vi "Receive Interface Status.vi"(8 "error in (no error)":errorcluster, 11 "Stream in":refnum<class "Stream.lvclass">) -> (0 "error out":errorcluster, 3 "Stream out":refnum<class "Stream.lvclass">)   [LabVIEW 2018, in "Stream.lvclass"]
uses:
  Stream.lvclass
  Interface/Interface.lvclass
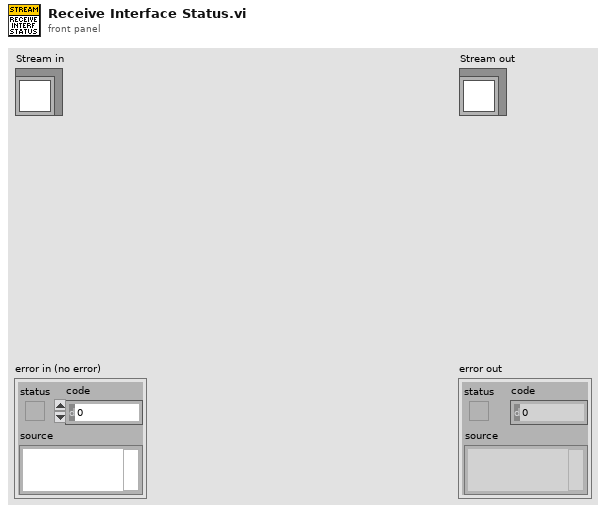
[diagram p1: front panel]
types:
  T1 = cluster{"Current Temperature":i16, "Temperatue Status":string}
  T2 = cluster{"Initialization":bool, "Serial Number":u16}
  T3 = cluster{"Exposure Time":sgl, "Pre-amp gain":u8, "Readout Rate":u8, "EM Mode":u8, "EM Gain":u16, "Binning":u16, "Initial Line":u16, "Initial Cloumn":u16, "Final Line":u16, "Final Column":u16, "Kinetic Series Length":u32, "Shutter Mode":u8, "Cooler ON/OFF":u16, "Temperature":i8, "Image Name":string, "Image Path":string, "#Images":u32, "Trigger":u16}
  T4 = cluster{"CUBE_EXPOSURE_TIME":sgl, "CUBES_DONE":u16, "LAST_IMAGE_NAME":string, "DISK_SPACE":u16, "FRAMES_DONE":u16, "CCD_STATUS":string, "CURRENT_TEMPERATURE":i16, "TEMPERATURE_STATUS":string, "FRAME_EXPOSURE_TIME":u16, "CCD_ON_OFF":bool, "SERIAL_NUMBER":u16, "ACQUIRING":bool}
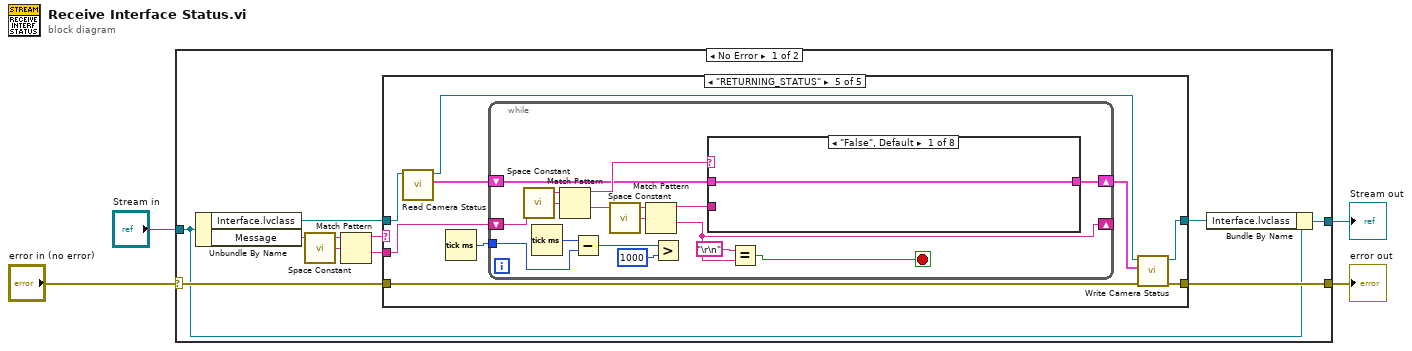
[diagram p0: block diagram]
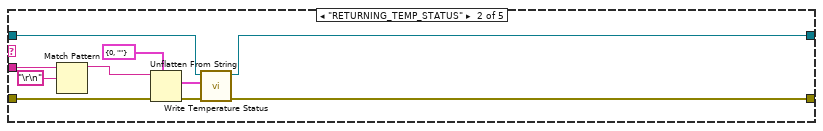
[diagram p3: hidden frame]
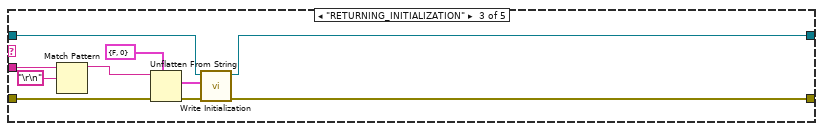
[diagram p4: hidden frame]
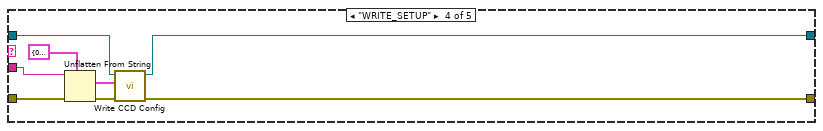
[diagram p5: hidden frame]
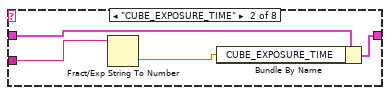
[diagram p6: hidden frame]
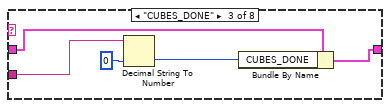
[diagram p7: hidden frame]
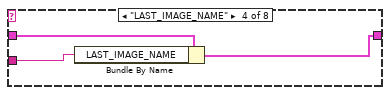
[diagram p8: hidden frame]
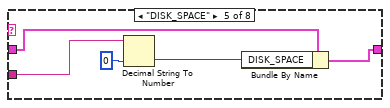
[diagram p9: hidden frame]
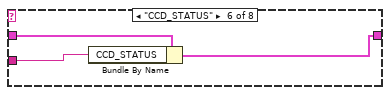
[diagram p10: hidden frame]
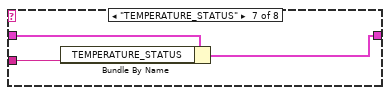
[diagram p11: hidden frame]
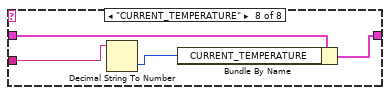
[diagram p12: hidden frame]
diagram:
  n1 = case shown="No Error" "error in (no error)" {
    selector: "error in (no error)" -> [w8 w98]
    tunnel: [w9 w98] -> w3
    tunnel: [w6 w97] -> w1
    tunnel: "Stream in" -> [w7 w97]
    frame No Error {
      n2 = Unbundle By Name(w7) -> ("Interface.lvclass"=w11:refnum<class "Interface.lvclass">, "Message"=w10:string)
      n3 = call <vilib>:"Space Constant.vi"() -> ("String"=w14:string)
      n4 = Match Pattern(string=w10, regular expression=w14) -> (before substring=w5:string, after substring=w13:string)  [unwired: 1 in, 2 out]
      n5 = case shown="\"RETURNING_STATUS\"" w5 {
        tunnel: w13 -> [_ w19 w28 w39 w45]
        tunnel: [w16 w26 w33 w41 w49] -> w12
        tunnel: w11 -> [w16 w25 w34 w40 w52]
        tunnel: [w15 w21 w32 w42 w48] -> w9
        tunnel: w8 -> [w15 w20 w31 w43 w47]
        frame "False", Default {
        }
        frame "RETURNING_TEMP_STATUS" {
          n6 = Match Pattern(string=w19, regular expression="\r\n") -> (before substring=w17:string)  [unwired: 1 in, 3 out]
          n7 = Unflatten From String(type=T1 {"Current Temperature"=0, "Temperatue Status"=""} ("Temperature Status"), binary string=w17, error in (no error)=w20) -> (value=w23:T1, error out=w24:errorcluster)  [unwired: 2 in, 1 out]
          n8 = call "Write Temperature Status.vi"("error in (no error)"=w24, "Temperature Status"=w23, "Interface in"=w25) -> ("error out"=w21:errorcluster, "Interface out"=w26:refnum<class "Interface.lvclass">)  [unwired: 7 in]
        }
        frame "RETURNING_INITIALIZATION" {
          n9 = Match Pattern(string=w28, regular expression="\r\n") -> (before substring=w27:string)  [unwired: 1 in, 3 out]
          n10 = Unflatten From String(type=T2 {"Initialization"=FALSE, "Serial Number"=0} ("Initialization"), binary string=w27, error in (no error)=w31) -> (value=w30:T2, error out=w36:errorcluster)  [unwired: 2 in, 1 out]
          n11 = call "Write Initialization.vi"("error in (no error)"=w36, "Initialization"=w30, "Interface in"=w34) -> ("error out"=w32:errorcluster, "Interface out"=w33:refnum<class "Interface.lvclass">)  [unwired: 7 in]
        }
        frame "WRITE_SETUP" {
          n12 = Unflatten From String(type=T3 {"Exposure Time"=0.0, "Pre-amp gain"=0, "Readout Rate"=0, "EM Mode"=0, "EM Gain"=0, "Binning"=0, "Initial Line"=0, "Initial Cloumn"=0, "Final Line"=0, "Final Column"=0, "Kinetic Series Length"=0, "Shutter Mode"=0, "Cooler ON/OFF"=0, "Temperature"=0, "Image Name"="", "Image Path"="", "#Images"=0, "Trigger"=0} ("CCD Config"), binary string=w39, error in (no error)=w43) -> (value=w38:T3, error out=w44:errorcluster)  [unwired: 2 in, 1 out]
          n13 = call "Write CCD Config.vi"("error in (no error)"=w44, "CCD Config"=w38, "Interface in"=w40) -> ("error out"=w42:errorcluster, "Interface out"=w41:refnum<class "Interface.lvclass">)  [unwired: 7 in]
        }
        frame "RETURNING_STATUS" {
          n14 = call "Read Camera Status.vi"("Interface in"=w52) -> ("Camera Status"=w50:T4, "Interface out"=w51:refnum<class "Interface.lvclass">)  [unwired: 8 in, 1 out]
          n15 = Tick Count (ms)() -> (millisecond timer value=w46:u32)
          n16 = while {
            shift-right: [w65] -> w53
            shift-left: w50 -> [w64]
            shift-right: [w60] -> _
            shift-left: w45 -> [w67]
            tunnel: w46 -> [w57]
            stop <- w54 stop-if-true
            n17 = call <vilib>:"Space Constant.vi"() -> ("String"=w68:string)
            n18 = Tick Count (ms)() -> (millisecond timer value=w58:u32)
            n19 = Match Pattern(string=w67, regular expression=w68) -> (before substring=w66:string, after substring=w62:string)  [unwired: 1 in, 2 out]
            n20 = Subtract(x=w58, y=w57) -> (x-y=w56:u32)
            n21 = call <vilib>:"Space Constant.vi"() -> ("String"=w63:string)
            n22 = Match Pattern(string=w62, regular expression=w63) -> (before substring=w61:string, after substring=w60:string)  [unwired: 1 in, 2 out]
            n23 = Greater?(x=w56, y=1000) -> ()  [unwired: 1 out]
            n24 = case shown="\"False\", Default" w66 {
              tunnel: [w69 w73 w78 w81 w86 w89 w92 w96] -> w65
              tunnel: w61 -> [_ w71 w76 w79 w83 w87 w90 w94]
              tunnel: w64 -> [w69 w72 w77 w80 w85 w88 w91 w95]
              frame "False", Default {
              }
              frame "CUBE_EXPOSURE_TIME" {
                n25 = Fract/Exp String To Number(string=w71) -> (number=w70:dbl)  [unwired: 3 in, 1 out]
                n26 = Bundle By Name(cluster=w72, "CUBE_EXPOSURE_TIME"=w70) -> (w73:T4)
              }
              frame "CUBES_DONE" {
                n27 = Decimal String To Number(string=w76, default (0L)=u16 0 ("default (0 I32)")) -> (number=w75:u16)  [unwired: 1 in, 1 out]
                n28 = Bundle By Name(cluster=w77, "CUBES_DONE"=w75) -> (w78:T4)
              }
              frame "LAST_IMAGE_NAME" {
                n29 = Bundle By Name(cluster=w80, "LAST_IMAGE_NAME"=w79) -> (w81:T4)
              }
              frame "DISK_SPACE" {
                n30 = Decimal String To Number(string=w83, default (0L)=u16 0 ("default (0 I32)")) -> (number=w84:u16)  [unwired: 1 in, 1 out]
                n31 = Bundle By Name(cluster=w85, "DISK_SPACE"=w84) -> (w86:T4)
              }
              frame "CCD_STATUS" {
                n32 = Bundle By Name(cluster=w88, "CCD_STATUS"=w87) -> (w89:T4)
              }
              frame "TEMPERATURE_STATUS" {
                n33 = Bundle By Name(cluster=w91, "TEMPERATURE_STATUS"=w90) -> (w92:T4)
              }
              frame "CURRENT_TEMPERATURE" {
                n34 = Decimal String To Number(string=w94) -> (number=w93:i32)  [unwired: 2 in, 1 out]
                n35 = Bundle By Name(cluster=w95, "CURRENT_TEMPERATURE"=w93) -> (w96:T4)
              }
            }
            n36 = Equal?(x="\r\n", y=w60) -> (x = y?=w54:bool)
          }
          n37 = call "Write Camera Status.vi"("error in (no error)"=w47, "Camera Status"=w53, "Interface in"=w51) -> ("error out"=w48:errorcluster, "Interface out"=w49:refnum<class "Interface.lvclass">)  [unwired: 7 in]
        }
      }
      n38 = Bundle By Name(cluster=w7, "Interface.lvclass"=w12) -> (w6:refnum<class "Stream.lvclass">)
    }
    frame Error {
    }
  }
  "error out" <- w3
  "Stream out" <- w1
